vi "UseCaseNode_Create.vi"(0 "reference":refnum<class "UseCaseNode.lvclass">, 5 "error in (no error)":errorcluster) -> (14 "reference out":refnum<class "UseCaseNode.lvclass">, 19 "error out":errorcluster)   [LabVIEW 2014, in "UseCaseNode.lvclass"]
doc: "Creates and initializes a new UseCaseNode object.\n\nThis object should be destroyed using a UseCaseNode destructor VI or a virtual base class destructor VI.\n\n[GOOP 2.1]"
uses:
  <resource>/Framework/Providers/Open_GDS/UML/UseCaseNode_class/UseCaseNode.lvclass
  <resource>/Framework/Providers/Open_GDS/UML/MultiLineString_class/SizeType.ctl
  <resource>/Framework/Providers/Open_GDS/UML/General/Rectangle/Rectangle Rectangle2D.ctl
  <resource>/Framework/Providers/Open_GDS/UML/MultiLineString_class/JustificationType.ctl
  <resource>/Framework/Providers/Open_GDS/UML/MultiLineString_class/MultiLineString.lvclass
  <resource>/Framework/Providers/Open_GDS/UML/RectangularNode_class/RectangularNode.lvclass
panel:
  # "The input reference should only\nbe wired when this method is called\nby a sub class constructor."
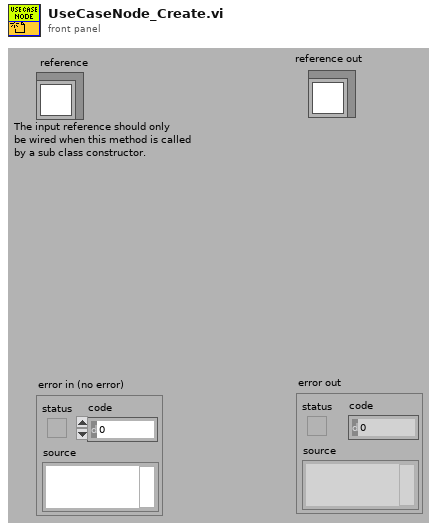
[diagram p1: front panel]
types:
  T1 = typedef "MultiLineString.lvclass/JustificationType.ctl" = enum16{"LEFT", "CENTER", "RIGHT"}
  T2 = typedef "Rectangle Rectangle2D.ctl" = cluster{"x":dbl, "y":dbl, "width":dbl, "height":dbl}
  T3 = typedef "MultiLineString.lvclass/SizeType.ctl" = enum16{"LARGE", "NORMAL", "SMALL"}
  T4 = typedef "UseCaseNode.lvclass/ObjectAttributes.ctl" = cluster{"name":refnum<class "MultiLineString.lvclass">, "DEFAULT_WIDTH":i32, "DEFAULT_HEIGHT":i32}
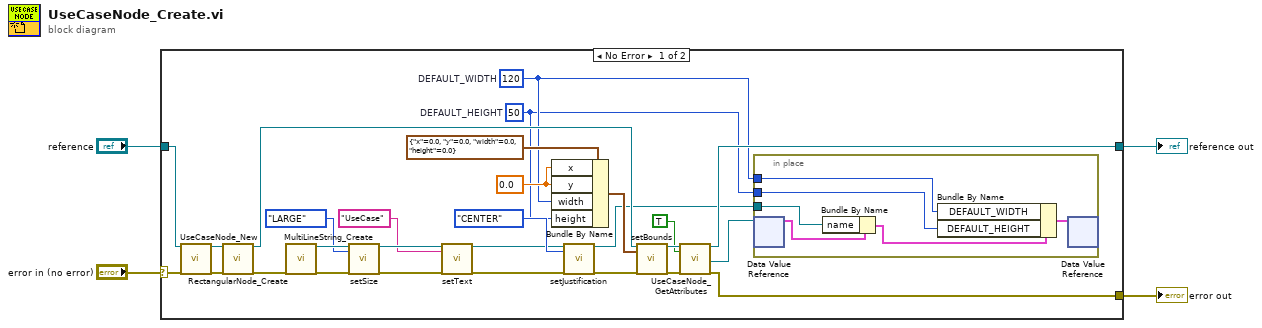
[diagram p0: block diagram]
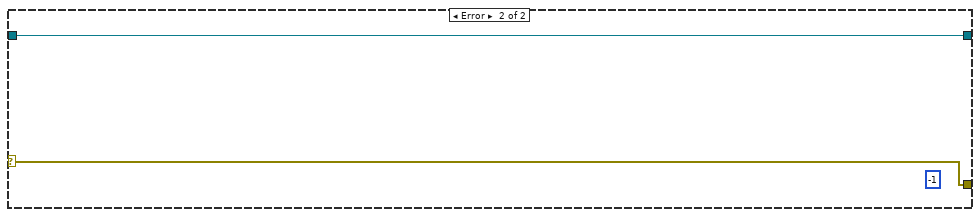
[diagram p2: hidden frame]
diagram:
  n1 = case shown="No Error" "error in (no error)" {
    selector: "error in (no error)" -> [w32 w40]
    tunnel: [w30 w39] -> w4
    tunnel: [w29 w40] -> w3
    tunnel: "reference" -> [w31 w39]
    frame No Error {
      w19 = 0.0 ("x")
      w5 = 50  # DEFAULT_HEIGHT
      w6 = 120  # DEFAULT_WIDTH
      n2 = call <resource>:"UseCaseNode_New.vi"("reference in"=w31, "error in (no error)"=w32) -> ("reference out"=w17:refnum<class "UseCaseNode.lvclass">, "error out"=w28:errorcluster)  [unwired: 2 in, 14 out]
      n3 = call <resource>:"RectangularNode_Create.vi"("reference"=w17, "error in (no error)"=w28) -> ("reference out"=w22:refnum<class "UseCaseNode.lvclass">, "error out"=w27:errorcluster)  [unwired: 1 in, 15 out]
      n4 = call <resource>:"MultiLineString_Create.vi"("error in (no error)"=w27) -> ("reference out"=w26:refnum<class "MultiLineString.lvclass">, "error out"=w25:errorcluster)  [unwired: 2 in, 15 out]
      n5 = call <resource>:"setSize.vi"("reference"=w26, "size"=SizeType."LARGE", "error in (no error)"=w25) -> ("reference out"=w15:refnum<class "MultiLineString.lvclass">, "error out"=w14:errorcluster)  [unwired: 15 out]
      n6 = call-dynamic "setText.vi"("reference"=w15, "text"="UseCase", "error in (no error)"=w14) -> ("reference out"=w11:refnum<class "MultiLineString.lvclass">, "error out"=w12:errorcluster)  [unwired: 15 in]
      n7 = Bundle By Name(cluster=T2 {"x"=0.0, "y"=0.0, "width"=0.0, "height"=0.0} ("bounds"), "x"=w19, "y"=w19, "width"=w6, "height"=w5) -> (w21:T2)
      n8 = call <resource>:"setJustification.vi"("reference"=w11, "justification"=JustificationType."CENTER", "error in (no error)"=w12) -> ("reference out"=w7:refnum<class "MultiLineString.lvclass">, "error out"=w18:errorcluster)  [unwired: 15 out]
      n9 = call-dynamic "setBounds.vi"("reference"=w22, "bounds"=w21, "error in (no error)"=w18) -> ("reference out"=w10:refnum<class "UseCaseNode.lvclass">, "error out"=w16:errorcluster)  [unwired: 15 in]
      n10 = call <resource>:"UseCaseNode_GetAttributes.vi"("reference in"=w10, "OnlyGetDvrReference(False)"=TRUE, "error in (no error)"=w16) -> ("reference out"=w30:refnum<class "UseCaseNode.lvclass">, "DataRef"=w8:refnum<data-value>, "error out"=w29:errorcluster)  [unwired: 13 in, 1 out]
      n11 = in-place {
        in-place-border: w7 -> [w37]
        in-place-border: w6 -> [w35]
        in-place-border: w5 -> [w34]
        n12 = in-place-dvr #1(w8) -> (w38:T4)  [unwired: 1 out]
        n13 = Bundle By Name(cluster=w38, "name"=w37) -> (w36:T4)
        n14 = Bundle By Name(cluster=w36, "DEFAULT_WIDTH"=w35, "DEFAULT_HEIGHT"=w34) -> (w33:T4)
        n15 = in-place-dvr #1(w33) -> ()  [unwired: 2 out]
      }
    }
    frame Error {
      (unwired) -1 ("Nr of open handles")
    }
  }
  "error out" <- w3
  "reference out" <- w4
